vi "Main.vi"(7 "log?":bool, 9 "Path Data Controller":path=path "/Users/baumann/Documents/SemesterProject1/TP_control_systems/MATLAB/dataRST.bin", 10 "Path Controller":path=path "/Users/baumann/Documents/SemesterProject1/TP_control_systems/C/src/TP2+TP3/rst.so") -> ()   [LabVIEW 2020]
uses:
  Qube/mode.ctl
  Qube/Qube.lvclass
panel:
  in  "mode":T1
  out "dt":dbl(graph)
  out "u":dbl(graph)
  in  "refgen":cluster{"Amplitude":dbl, "Period (ms)":dbl}
  out "error":errorcluster
  in  "stop":bool
  out "y + r":cluster{"y":dbl, "y":dbl}(graph)
  # "1) Set the pathCtrl to the location of your\n     controller (the shared object .so)\n2) Set the pathDataCtrl to the location of \n     the controller data from MATLAB\n3) Press the white arrow near the top-left\n     corner. \n4) You can eventually log the data by\npressing \"Record\"."
  # "Change the Amplitude and period value to see how your controller can track  steps."
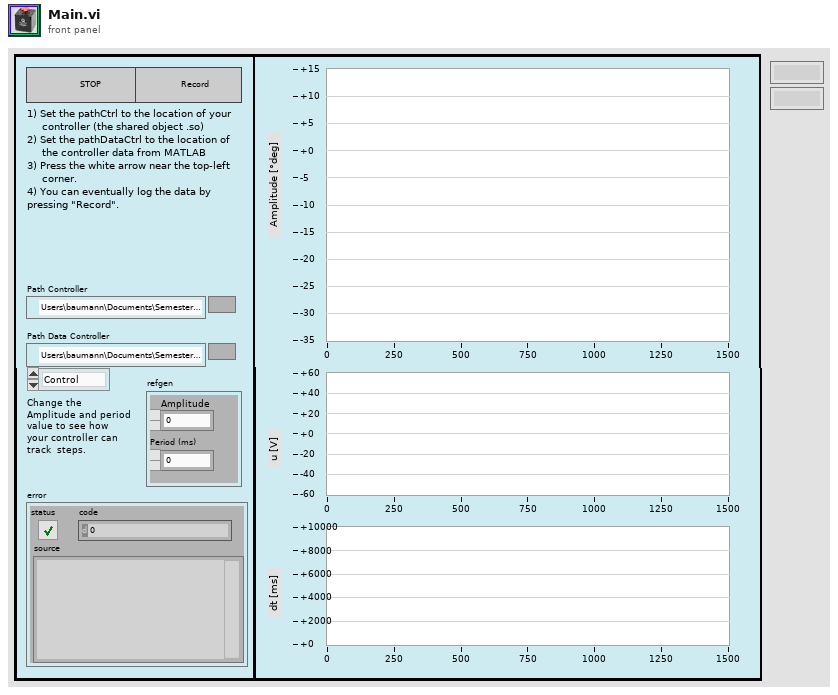
[diagram p1: front panel]
types:
  T1 = typedef "Qube.lvclass/mode.ctl" = enum16{"Control", "Identify"}
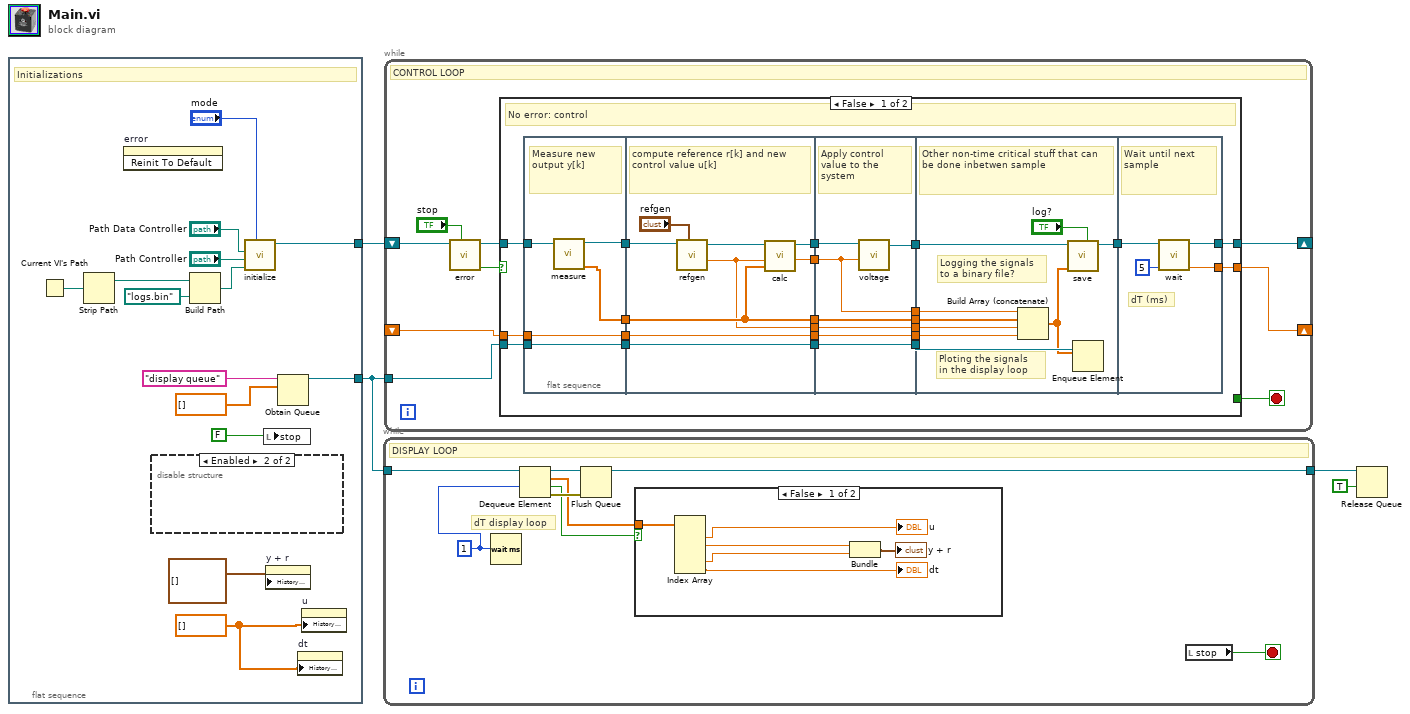
[diagram p0: block diagram]
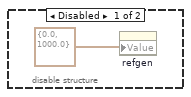
[diagram p3: hidden frame]
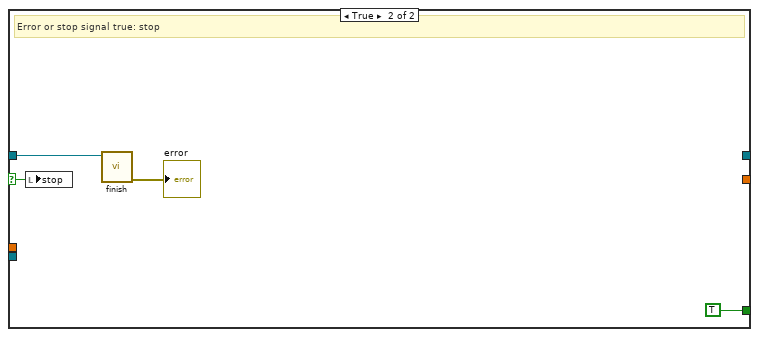
[diagram p4: hidden frame]
diagram:
  n1 = flat-sequence {
    tunnel: [w13] -> w4
    tunnel: [w18] -> w3
    frame #0 {
      w5 = dbl[] [] ("Waveform Chart")
      # "Initializations"
      n2 = Current VI's Path() -> (path=w12:path)
      n3 = Strip Path(path=w12) -> (stripped path=w11:path)  [unwired: 1 out]
      n4 = invoke on="error" class="Clust (strict)" method="Reinit To Default"() -> ()  [unwired: 3 in, 3 out]
      n5 = disable-structure shown="Enabled" {
        frame Disabled {
          n6 = property on="refgen" class="Clust (strict)"("Value"=cluster{"slope":dbl, "period":dbl} {"slope"=0.0, "period"=1000.0} ("refgen")) -> ()  [unwired: 2 in, 2 out]
        }
        frame Enabled {
        }
      }
      n7 = Build Path(base path=w11, name or relative path=path "logs.bin") -> (appended path=w9:path)
      n8 = call "initialize.vi"("mode"="mode", "log path"=w9, "pathCtrl"="Path Controller", "pathDataCtrl"="Path Data Controller") -> ("Qube"=w13:refnum<class "Qube.lvclass">)  [unwired: 7 in]
      n9 = local write "stop"(FALSE ("stop")) -> ()
      n10 = property on="y + r" class="WFChart (strict)"("History Data"=cluster{"y":dbl, "y":dbl}[] []) -> ()  [unwired: 2 in, 2 out]
      n11 = Obtain Queue(name (unnamed)="display queue", element data type=dbl[] [] ("y")) -> (queue out=w18:refnum<queue>)  [unwired: 3 in, 2 out]
      n12 = property on="dt" class="WFChart (strict)"("History Data"=w5) -> ()  [unwired: 2 in, 2 out]
      n13 = property on="u" class="WFChart (strict)"("History Data"=w5) -> ()  [unwired: 2 in, 2 out]
    }
  }
  n14 = while {
    tunnel: w3 -> [w26]
    tunnel: [w24] -> w1
    stop <- w27 stop-if-true
    w22 = u32 1 ("Ts")
    # "dT display loop"
    # "DISPLAY LOOP"
    n15 = Wait (ms)(milliseconds to wait=w22) -> ()  [unwired: 1 out]
    n16 = Dequeue Element(queue=w26, timeout in ms (-1)=w22) -> (queue out=w25:refnum<queue>, element=w20:dbl[], timed out?=w21:bool, error out=w23:errorcluster)  [unwired: 1 in]
    n17 = Flush Queue(queue=w25, error in (no error)=w23) -> (queue out=w24:refnum<queue>)  [unwired: 2 out]
    n18 = case shown="False" w21 {
      tunnel: w20 -> [w32 _]
      frame False {
        n19 = Index Array(array=w32) -> (element #1=→"u":dbl, element #2=w31:dbl, element #4=w28:dbl, element #5=→"dt":dbl)  [unwired: 5 in, 1 out]
        n20 = Bundle("y"=w31, "y"=w28) -> (→"y + r":cluster{"y":dbl, "y":dbl})  [unwired: 1 in]
      }
      frame True {
      }
    }
    n21 = local read "stop"() -> (w27:bool)
  }
  n22 = while {
    shift-right: [w41] -> _
    shift-left: w4 -> [w35]
    tunnel: w3 -> [w40]
    shift-right: [w39] -> _
    shift-left: _ -> [w34]
    stop <- w42 stop-if-true
    # "CONTROL LOOP"
    n23 = call "error.vi"("stop"="stop", "Qube"=w35) -> ("abort?"=w37:bool, "Qube"=w38:refnum<class "Qube.lvclass">)  [unwired: 8 in]
    n24 = case shown="False" w37 {
      selector: w37 -> [_ w100]
      tunnel: w38 -> [w48 w101]
      tunnel: [_ TRUE] -> w42
      tunnel: [w61 _] -> w41
      tunnel: w40 -> [w58 _]
      tunnel: [w53 _] -> w39
      tunnel: w34 -> [w54 _]
      frame False {
        # "No error: control"
        n25 = flat-sequence {
          tunnel: w54 -> [w68]
          tunnel: w58 -> [w69]
          tunnel: [w66] -> w52
          tunnel: [w65] -> w51
          tunnel: [w69] -> w50
          tunnel: [w68] -> w49
          tunnel: w48 -> [w67]
          tunnel: [w75] -> w60
          tunnel: [w73] -> w59
          tunnel: [w78] -> w56
          tunnel: w52 -> [w77]
          tunnel: w51 -> [w73]
          tunnel: w50 -> [w78]
          tunnel: w49 -> [w71]
          tunnel: [w72] -> w46
          tunnel: [w71] -> w45
          tunnel: [w70] -> w43
          tunnel: [w85] -> w64
          tunnel: [w84] -> w62
          tunnel: w60 -> [w82]
          tunnel: w59 -> [w84]
          tunnel: [w83] -> w57
          tunnel: w56 -> [w83]
          tunnel: [w79] -> w55
          tunnel: [w81] -> w47
          tunnel: w46 -> [w81]
          tunnel: w45 -> [w80]
          tunnel: [w80] -> w44
          tunnel: w43 -> [w79]
          tunnel: w64 -> [w89]
          tunnel: [w94] -> w63
          tunnel: w62 -> [w93]
          tunnel: w57 -> [w91]
          tunnel: w55 -> [w88]
          tunnel: w47 -> [w87]
          tunnel: w44 -> [w86]
          tunnel: [w97] -> w61
          tunnel: w63 -> [w98]
          tunnel: [w95] -> w53
          frame #0 {
            # "Measure new output y[k]"
            n26 = call "measure.vi"("Qube"=w67) -> ("y"=w65:dbl[], "Qube"=w66:refnum<class "Qube.lvclass">)  [unwired: 8 in, 1 out]
          }
          frame #1 {
            # "compute reference r[k] and new control value u[k]"
            n27 = call "refgen.vi"("refgen"="refgen", "Qube"=w77) -> ("r"=w72:dbl, "Qube"=w76:refnum<class "Qube.lvclass">)  [unwired: 8 in]
            n28 = call "calc.vi"("y"=w73, "r"=w72, "Qube"=w76) -> ("u"=w70:dbl, "Qube"=w75:refnum<class "Qube.lvclass">)  [unwired: 7 in]
          }
          frame #2 {
            # "Apply control \nvalue to the system"
            n29 = call "voltage.vi"("u"=w79, "Qube"=w82) -> ("Qube"=w85:refnum<class "Qube.lvclass">)  [unwired: 9 in]
          }
          frame #3 {
            # "Ploting the signals\nin the display loop"
            # "Logging the signals to a binary file?"
            # "Other non-time critical stuff that can be done inbetwen sample"
            n30 = Build Array (concatenate)(w88, w93, w87, w86) -> (w90:dbl[])
            n31 = call "save.vi"("log?"="log?", "data"=w90, "Qube"=w89) -> ("Qube"=w94:refnum<class "Qube.lvclass">)  [unwired: 8 in]
            n32 = Enqueue Element(queue=w91, element=w90) -> ()  [unwired: 2 in, 3 out]
          }
          frame #4 {
            # "dT (ms)"
            # "Wait until next sample"
            n33 = call "wait.vi"("Ts (ms)"=u32 5, "Qube"=w98) -> ("dt"=w95:dbl, "Qube"=w97:refnum<class "Qube.lvclass">)  [unwired: 8 in]
          }
        }
      }
      frame True {
        # "Error or stop signal true: stop"
        n34 = local write "stop"(w100) -> ()
        n35 = call "finish.vi"("ActiveSuspension.lvclass"=w101) -> ("error out"=→"error":errorcluster)  [unwired: 10 in]
      }
    }
  }
  n36 = Release Queue(queue=w1, force destroy? (F)=TRUE) -> ()  [unwired: 1 in, 3 out]
